vi "Elapsed Timer FGV.vi"(8 "error in (no error)":errorcluster, 10 "Time to count down to (s)":dbl, 11 "Command":T1) -> (0 "error out":errorcluster, 1 "Elapsed?":bool, 2 "Current Elapsed time (s)":dbl)   [LabVIEW 2018]
doc: "This VI acts as a timer to track the elapsed time.\n\n\n(Nimble Focus Consulting 2016)"
uses:
  Enum - Programme Checker Machine State Typedef.ctl
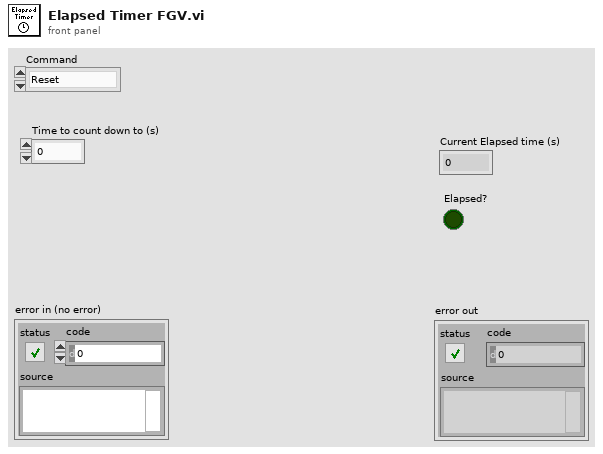
[diagram p1: front panel]
types:
  T1 = typedef "Enum - Programme Checker Machine State Typedef.ctl" = enum16{"Reset", "Check Elapsed Time"}
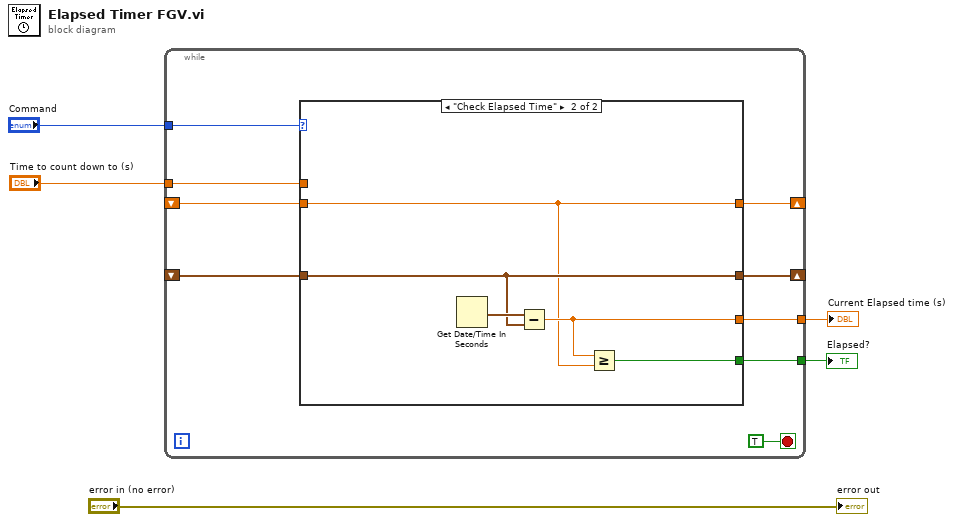
[diagram p0: block diagram]
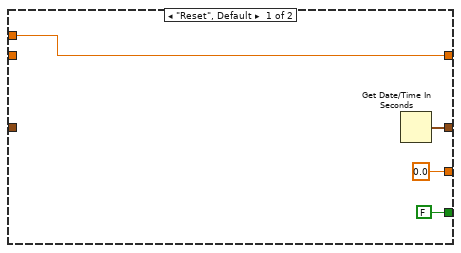
[diagram p2: hidden frame]
diagram:
  n1 = while {
    tunnel: "Command" -> [w13]
    tunnel: "Time to count down to (s)" -> [w12]
    shift-right: [w11] -> _
    shift-left: _ -> [w10]
    shift-right: [w9] -> _
    shift-left: _ -> [w8]
    tunnel: [w7] -> w2
    tunnel: [w6] -> w1
    stop <- TRUE stop-if-true
    n2 = case shown="\"Check Elapsed Time\"" w13 {
      tunnel: w12 -> [w18 _]
      tunnel: [w18 w20] -> w11
      tunnel: w10 -> [_ w20]
      tunnel: [w17 w22] -> w9
      tunnel: w8 -> [_ w22]
      tunnel: [0.0 w21] -> w7
      tunnel: [FALSE w19] -> w6
      frame "Reset", Default {
        n3 = Get Date/Time In Seconds() -> (seconds since 1Jan1904=w17:timestamp)
      }
      frame "Check Elapsed Time" {
        n4 = Get Date/Time In Seconds() -> (seconds since 1Jan1904=w23:timestamp)
        n5 = Subtract(x=w23, y=w22) -> (x-y=w21:dbl)
        n6 = Greater Or Equal?(x=w21, y=w20) -> (x >= y?=w19:bool)
      }
    }
  }
  "Elapsed?" <- w1
  "Current Elapsed time (s)" <- w2
  "error out" <- "error in (no error)"
